vi "TOPAZ.vi"() -> ()   [LabVIEW 2018]
uses:
  <vilib>/Instr/_visa.llb/VISA Configure Serial Port (Instr).vi
panel:
  in  "Ослабление, дБ":ext format="%.2p"
  in  "Команды":T1(ring)
  in  "Длины волн, нм":enum16{"850", "1300", "1310", "1550"}(ring)
  out "return count 2":u32
  out "error out":errorcluster
  in  "error in (no error)":errorcluster
  out "return count":u32
  in  "milliseconds to wait":u32=2000
  in  "stop":bool
  in  "COM - порт":refnum<visa-resource-name>="COM14"
  in  "Текущее\nослабление? (дБ)":bool
  out "Ответ:":string
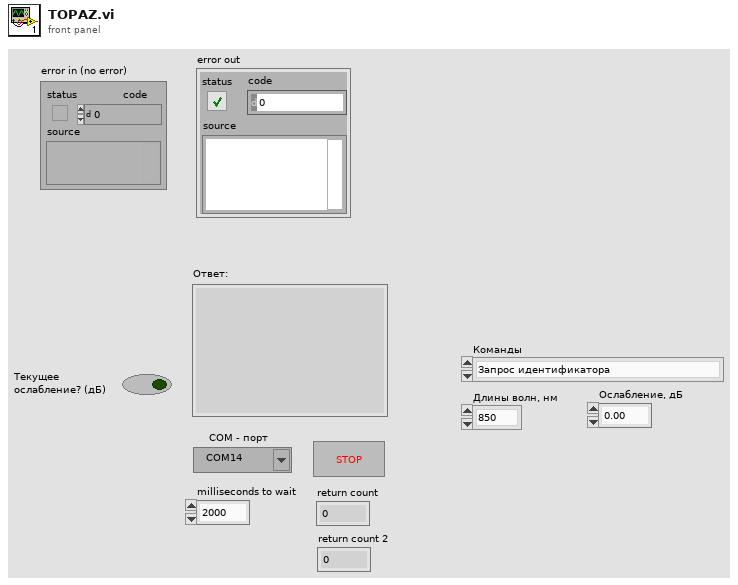
[diagram p1: front panel]
types:
  T1 = enum16{"Запрос идентификатора", "Запрос доступных длин волн, (нм)", "Запрос установленной длины волны, (нм)", "Запрос установленного ослабления, (дБ)", "Установка длины волны, (нм)", "Установка ослабления, (дБ)"}
  T2 = enum16{"Запрос идентификатора", "Запрос доступных длин волн, (нм)", "Запрос длины волы, (нм)", "Запрос ослабления, (дБ)", "Установка длины волны, (нм)", "Установка ослабления, (дБ)"}
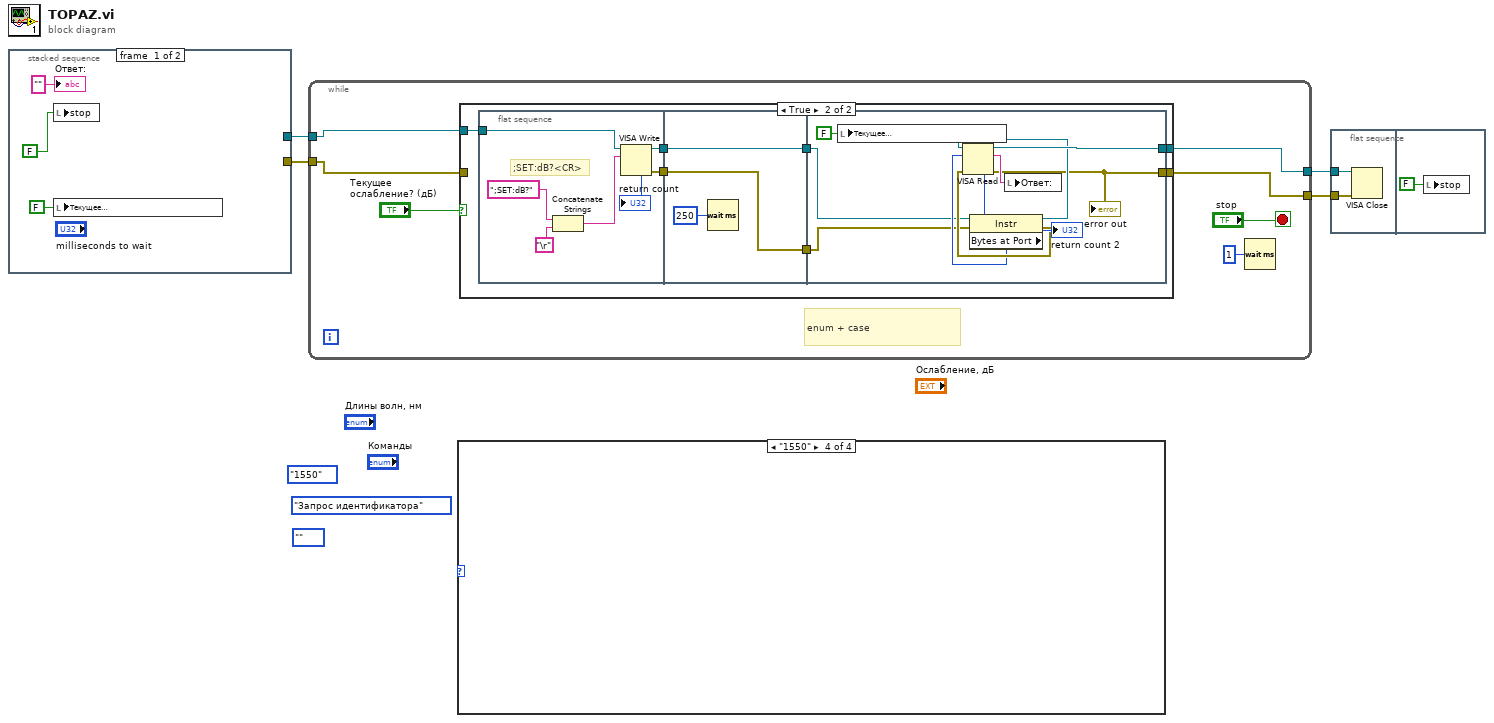
[diagram p0: block diagram]
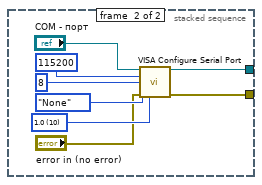
[diagram p5: hidden frame]
diagram:
  (unwired) enum16{""}.""
  (unwired) T2."Запрос идентификатора"
  (unwired) enum16{"850", "1300", "1310", "1550"}."1550"
  n1 = stacked-sequence {
    tunnel: [_ w10] -> w2
    tunnel: [_ w8] -> w1
    frame #0 {
      n2 = local write "stop"(FALSE ("stop")) -> ()
      n3 = local write "Текущее\nослабление? (дБ)"(FALSE ("Текущее\nослабление? (дБ)")) -> ()
      "Ответ:" <- "" ("Ответ:")
    }
    frame #1 {
      w12 = u16 10 items=["1.0"=10, "1.5"=15, "2.0"=20] ("stop bits (10: 1 bit)")
      n4 = call-poly "VISA Configure Serial Port"("VISA resource name"="COM - порт", "baud rate (9600)"=u32 115200, "data bits (8)"=u16 8, "parity (0:none)"=enum16{"None", "Odd", "Even", "Mark", "Space"}."None", "error in (no error)"="error in (no error)", "stop bits (10: 1 bit)"=w12) -> ("VISA resource name out"=w10:refnum<visa-resource-name>, "error out"=w8:errorcluster)  [unwired: 8 in]
    }
  }
  n5 = while {
    tunnel: [w20] -> w4
    tunnel: [w19] -> w3
    tunnel: w2 -> [w18]
    tunnel: w1 -> [w17]
    stop <- "stop" stop-if-true
    # "enum + case"
    n6 = case shown="True" "Текущее\nослабление? (дБ)" {
      tunnel: [w24 w29] -> w20
      tunnel: [w23 w26] -> w19
      tunnel: w18 -> [w24 w25]
      tunnel: w17 -> [w23 _]
      frame False {
      }
      frame True {
        n7 = flat-sequence {
          tunnel: [w38] -> w30
          tunnel: [w36] -> w27
          tunnel: w25 -> [w35]
          tunnel: [w41] -> w31
          tunnel: w30 -> [w41]
          tunnel: [w40] -> w28
          tunnel: w27 -> [w40]
          tunnel: w31 -> [w44]
          tunnel: [w50] -> w29
          tunnel: w28 -> [w43]
          tunnel: [w45] -> w26
          frame #0 {
            # ";SET:dB?<CR>"
            n8 = Concatenate Strings(";SET:dB?", "\r") -> (w33:string)
            n9 = VISA Write(VISA resource name=w35, write buffer=w33) -> (VISA resource name out=w38:refnum<visa-resource-name>, return count=→"return count":u32, error out=w36:errorcluster)  [unwired: 1 in]
          }
          frame #1 {
            n10 = Wait (ms)(milliseconds to wait=u32 250 ("milliseconds to wait 2")) -> ()  [unwired: 1 out]
          }
          frame #2 {
            n11 = local write "Текущее\nослабление? (дБ)"(FALSE ("Текущее\nослабление? (дБ)")) -> ()
            n12 = property class="Instr"(reference=w44, error in=w43) -> (reference out=w48:refnum<visa-resource-name>, error out=w47:errorcluster, "Bytes at Port"=w46:u32)
            n13 = VISA Read(VISA resource name=w48, byte count=w46, error in (no error)=w47) -> (VISA resource name out=w50:refnum<visa-resource-name>, read buffer=w51:string, return count=→"return count 2":u32, error out=w45:errorcluster)
            "error out" <- w45
            n14 = local write "Ответ:"(w51) -> ()
          }
        }
      }
    }
    n15 = Wait (ms)(milliseconds to wait=u32 1) -> ()  [unwired: 1 out]
  }
  n16 = case shown="\"1550\"" {
    selector: _ -> [_ _ _ _]
    frame "850" {
    }
    frame "1300" {
    }
    frame "1310" {
    }
    frame "1550" {
    }
  }
  n17 = flat-sequence {
    tunnel: w4 -> [w53]
    tunnel: w3 -> [w52]
    frame #0 {
      n18 = VISA Close(VISA resource name=w53, error in (no error)=w52) -> ()  [unwired: 1 out]
    }
    frame #1 {
      n19 = local write "stop"(FALSE ("stop")) -> ()
    }
  }
